vi "CTRE_LibraryCall_ErrorHandle.vi"(8 "error in":errorcluster, 10 "DeviceType":string="Error occurred at ") -> (0 "error out":errorcluster)   [LabVIEW 2017]
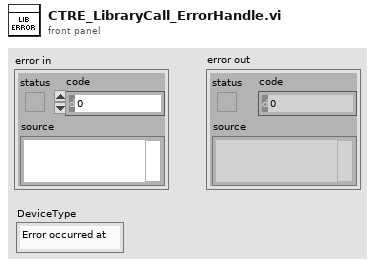
[diagram p1: front panel]
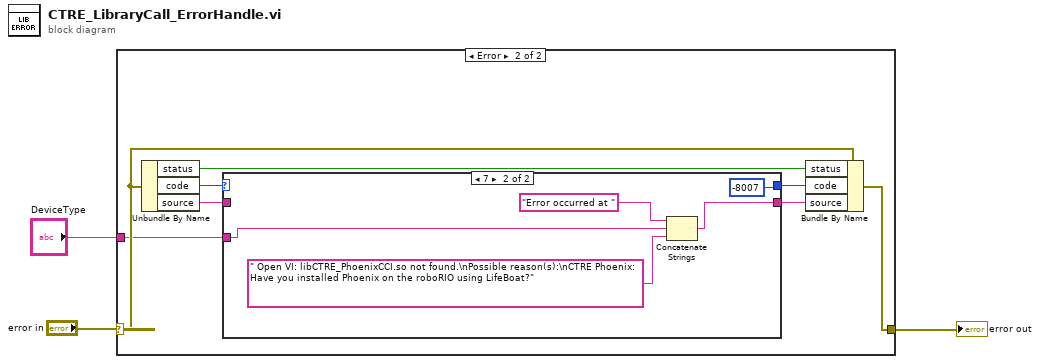
[diagram p0: block diagram]
diagram:
  n1 = case shown="Error" "error in" {
    selector: "error in" -> [w4 w12]
    tunnel: [w4 w11] -> w2
    tunnel: "DeviceType" -> [_ w5]
    frame No Error {
    }
    frame Error {
      n2 = Unbundle By Name(w12) -> ("status"=w10:bool, "code"=w9:i32, "source"=w8:string)
      n3 = case shown="7" w9 {
        selector: w9 -> [w13 _]
        tunnel: w8 -> [w14 _]
        tunnel: [w14 w18] -> w7
        tunnel: [w13 -8007 ("code")] -> w6
        tunnel: w5 -> [_ w16]
        frame 0, Default {
        }
        frame 7 {
          n4 = Concatenate Strings("Error occurred at " ("source"), w16, " Open VI: libCTRE_PhoenixCCI.so not found.\nPossible reason(s):\nCTRE Phoenix: Have you installed Phoenix on the roboRIO using LifeBoat?" ("string")) -> (w18:string)
        }
      }
      n5 = Bundle By Name(cluster=w12, "status"=w10, "code"=w6, "source"=w7) -> (w11:errorcluster)
    }
  }
  "error out" <- w2
